vi "ResizeObjectsinPane.vi"(8 "error in (no error)":errorcluster, 10 "PaneRef":refnum<vi>, 11 "PentaPanesGUI in":refnum<class "PentaPanes.lvclass">) -> (0 "error out":errorcluster, 3 "PentaPanesGUI out":refnum<class "PentaPanes.lvclass">)   [LabVIEW 2022 SP3, in "PentaPanesLibrary.lvlib" / "PentaPanes.lvclass"]
doc: "This VI resizes all registered control contained in the PaneRef pane. \n\nPaneRef - a reference to the pane"
uses:
  PentaPanes.lvclass
  PentaPanes.lvclass/PentaPanes.ctl
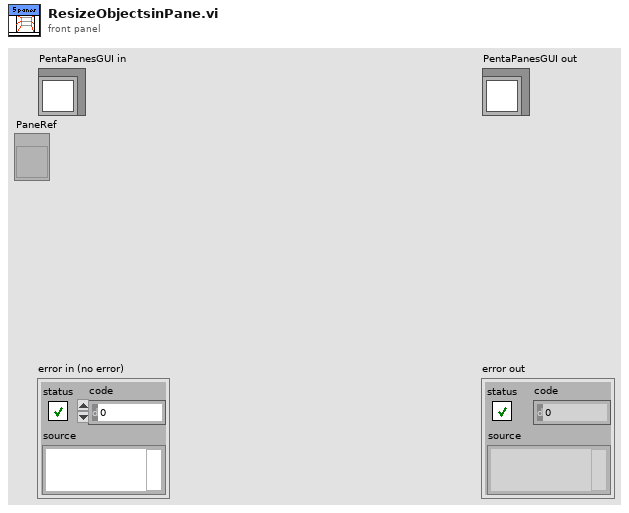
[diagram p1: front panel]
types:
  T1 = typedef "PentaPanesLibrary.lvlib/PentaPanes.lvclass/ResizableObject.ctl" = cluster{"generic class reference":refnum<vi>, "Label out":string, "Adjust":u16, "Borders":T2, "Minimal":T3, "Class Name out":string, "Class ID out":u32, "Owning Pane out":refnum<vi>, "Borders in Percent(T) or Pixels (F)":bool, "Invisible?":bool, "Force Aspect Ratio?":bool}
  T2 = typedef "PentaPanesLibrary.lvlib/PentaPanes.lvclass/BordersCluster.ctl" = cluster{"Left":i32, "Top":i32, "Right":i32, "Bottom":i32}
  T3 = typedef "LVBoundsTypeDef.ctl" = cluster{"Width":i32, "Height":i32}
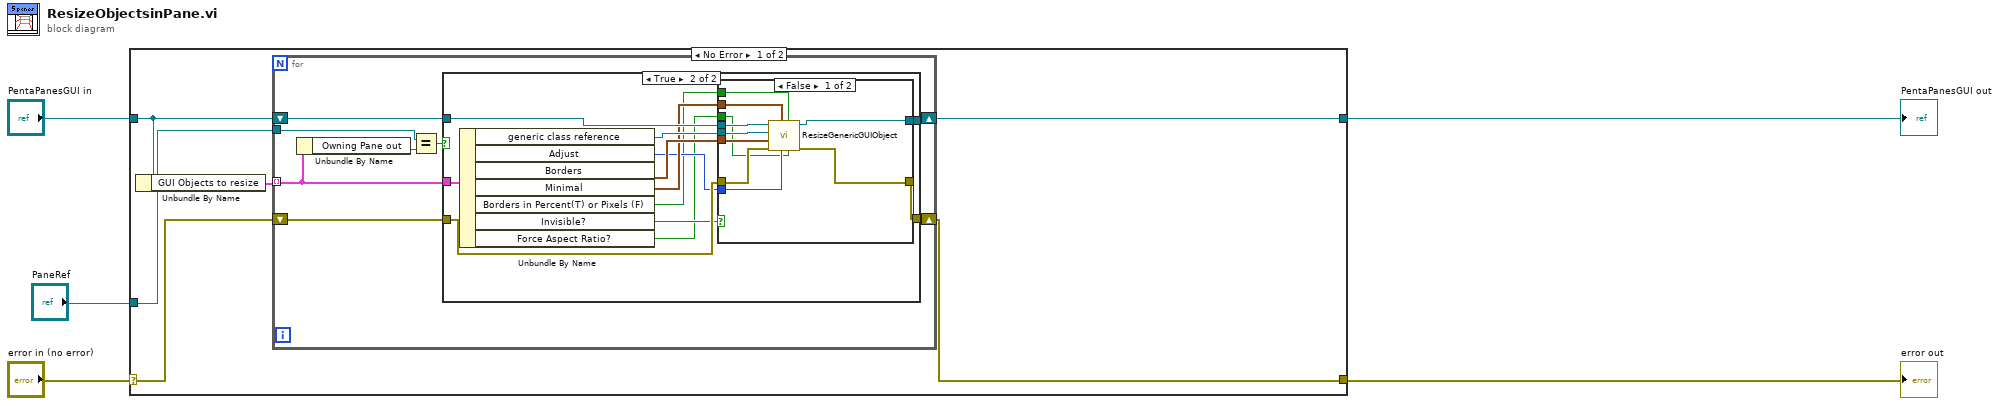
[diagram p0: block diagram]
diagram:
  n1 = case shown="No Error" "error in (no error)" {
    selector: "error in (no error)" -> [w7 w47]
    tunnel: [w6 w47] -> w4
    tunnel: [w11 w46] -> w2
    tunnel: "PentaPanesGUI in" -> [w9 w46]
    tunnel: "PaneRef" -> [w10 _]
    frame No Error {
      n2 = Unbundle By Name(w9) -> ("GUI Objects to resize"=w8:T1[])
      n3 = for {
        shift-right: [w18] -> w11
        shift-left: w9 -> [w19]
        shift-right: [w16] -> w6
        shift-left: w7 -> [w17]
        tunnel: w8 -> [w15] mode=indexing
        tunnel: w10 -> [w13]
        n4 = Unbundle By Name(w15) -> ("Owning Pane out"=w14:refnum<vi>)
        n5 = Equal?(x=w13, y=w14) -> (x = y?=w12:bool)
        n6 = case shown="True" w12 {
          tunnel: w19 -> [w21 w33]
          tunnel: [w21 w32] -> w18
          tunnel: w17 -> [w20 w31]
          tunnel: [w20 w30] -> w16
          tunnel: w15 -> [_ w22]
          frame False {
          }
          frame True {
            n7 = Unbundle By Name(w22) -> ("generic class reference"=w29:refnum<vi>, "Adjust"=w26:u16, "Borders"=w28:T2, "Minimal"=w27:T3, "Borders in Percent(T) or Pixels (F)"=w25:bool, "Invisible?"=w24:bool, "Force Aspect Ratio?"=w23:bool)
            n8 = case shown="False" w24 {
              tunnel: w33 -> [w43 w45]
              tunnel: [w42 w45] -> w32
              tunnel: w31 -> [w41 w44]
              tunnel: [w40 w44] -> w30
              tunnel: w29 -> [w39 _]
              tunnel: w28 -> [w38 _]
              tunnel: w27 -> [w37 _]
              tunnel: w26 -> [w36 _]
              tunnel: w25 -> [w35 _]
              tunnel: w23 -> [w34 _]
              frame False {
                n9 = call-dynamic "ResizeGenericGUIObject.vi"("Force Aspect Ratio?"=w34, "Borders in Percent(T) or Pixels (F)"=w35, "Adjust"=w36, "Minimal"=w37, "error in (no error)"=w41, "Borders"=w38, "generic class reference"=w39, "PentaPanesGUI in"=w43) -> ("error out"=w40:errorcluster, "PentaPanesGUI out"=w42:refnum<class "PentaPanes.lvclass">)  [unwired: 1 in, 1 out]
              }
              frame True {
              }
            }
          }
        }
      }
    }
    frame Error {
    }
  }
  "error out" <- w4
  "PentaPanesGUI out" <- w2
